vi "Fail.vi"(8 "error in (no error)":errorcluster, 11 "reference in":refnum<class "Test_Flux_Capacitor.lvclass">) -> (0 "error out":errorcluster, 3 "reference in":refnum<class "Test_Flux_Capacitor.lvclass">)   [LabVIEW 2022 SP3, in "Test_Flux_Capacitor.lvlib" / "Test_Flux_Capacitor.lvclass"]
uses:
  Test_Flux_Capacitor.lvclass
  Components/PSU_Base.lvlibp/PSU_Base.lvclass
  Components/SwitchBase.lvlibp/SwitchBase.lvclass
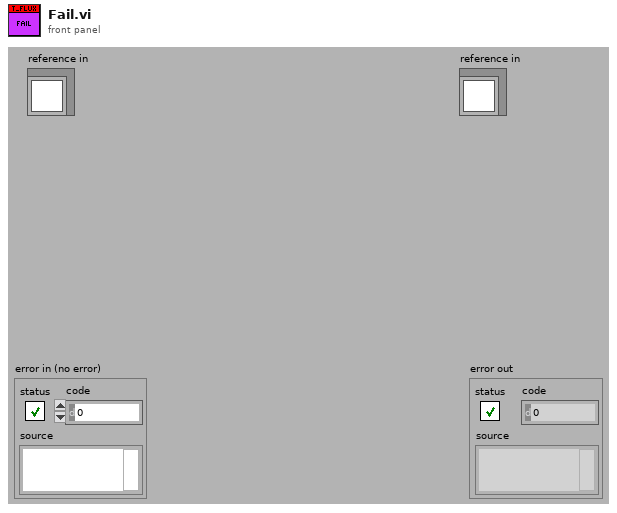
[diagram p1: front panel]
types:
  T1 = typedef "Test_Flux_Capacitor.lvlib/Test_Flux_Capacitor.lvclass/ObjectAttributes.ctl" = cluster{"Config":T2, "DMM":refnum<class "DMM_Keysight_34980A.lvclass">, "LCR":refnum<class "LCR_BK891.lvclass">, "PSU":refnum<class "PSU_Base.lvclass">, "Switch_Manager":refnum<class "SwitchBase.lvclass">, "FRAM":string, "Flux_Capacitor":refnum<class "Flux_Capacitor.lvclass">, "Frequency_Counter":refnum<class "Frequency_Counter_Base.lvclass">, "JTAG":refnum<class "JTAG_Base.lvclass">}
  T2 = typedef "Test_Flux_Capacitor.lvlib/Test_Flux_Capacitor.lvclass/Config.ctl" = cluster{"default":string}
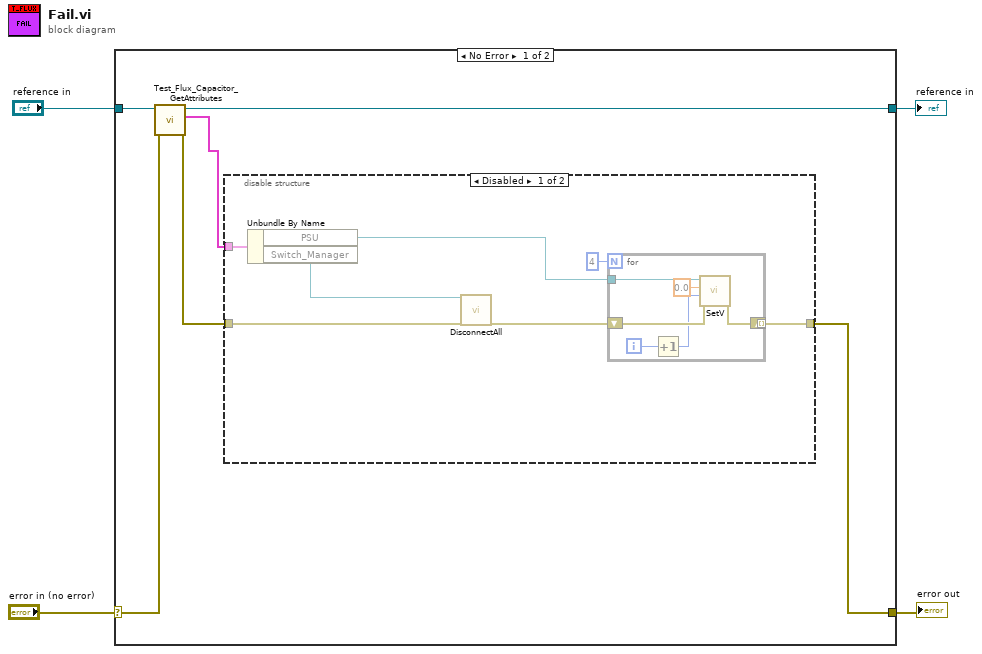
[diagram p0: block diagram]
diagram:
  n1 = case shown="No Error" "error in (no error)" {
    selector: "error in (no error)" -> [w10 w25]
    tunnel: [w5 w25] -> w3
    tunnel: [w8 w24] -> w1
    tunnel: "reference in" -> [w9 w24]
    frame No Error {
      n2 = call "Test_Flux_Capacitor_GetAttributes.vi"("error in (no error)"=w10, "reference in"=w9) -> ("error out"=w6:errorcluster, "Data"=w7:T1, "reference out"=w8:refnum<class "Test_Flux_Capacitor.lvclass">)  [unwired: 6 in, 1 out]
      n3 = disable-structure shown="Disabled" {
        disable-tunnel: w7 -> [w13 _]
        disable-tunnel: w6 -> [w12 _]
        disable-tunnel: [w11 _] -> w5
        frame Disabled {
          n4 = Unbundle By Name(w13) -> ("PSU"=w16:refnum<class "PSU_Base.lvclass">, "Switch_Manager"=w17:refnum<class "SwitchBase.lvclass">)
          n5 = call-dynamic "DisconnectAll.vi"("reference in"=w17, "error in (no error)"=w12) -> ("error out"=w14:errorcluster)  [unwired: 16 in, 1 out]
          n6 = for {
            N: 4 -> [_]
            tunnel: w16 -> [w23]
            shift-right: [w18] -> w11
            shift-left: w14 -> [w22]
            tunnel: [w18] -> _ mode=indexing
            i -> [w21]
            n7 = Increment(x=w21) -> (x+1=w20:i32)
            n8 = call-dynamic "SetV.vi"("error in (no error)"=w22, "Chan"=w20, "V"=0.0, "reference in"=w23) -> ("error out"=w18:errorcluster)  [unwired: 6 in, 1 out]
          }
        }
        frame Enabled {
        }
      }
    }
    frame Error {
    }
  }
  "error out" <- w3
  "reference in" <- w1
